vi "Apply Tombstone Target.vi"   [LabVIEW 2018, in "Toolkit.lvlib" / "Tests.lvlib"]
uses:
  Tests.lvlib
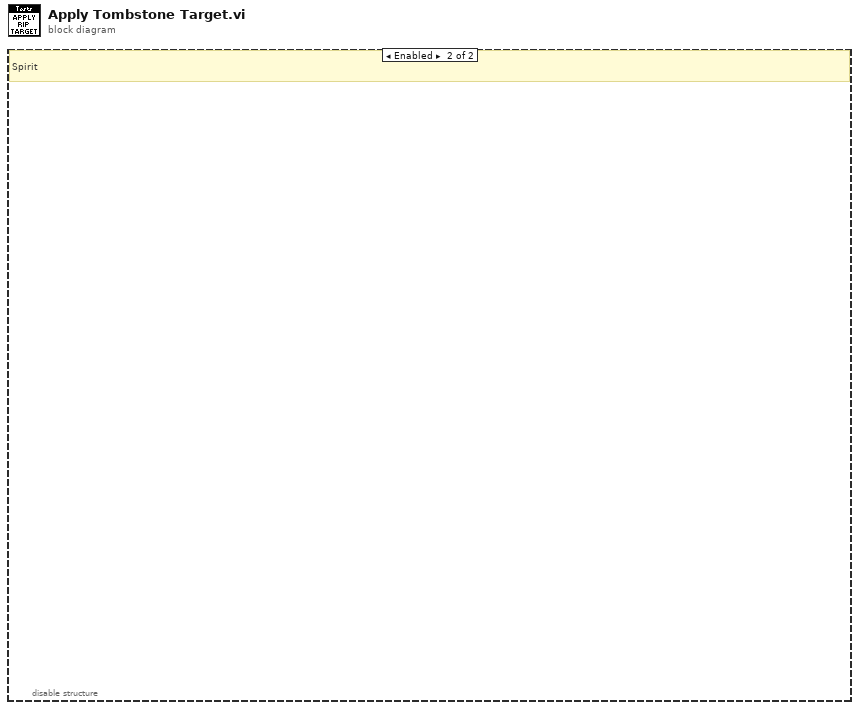
[diagram p0: block diagram]
diagram:
  n1 = disable-structure shown="Enabled" {
    frame Disabled {
      # "Corpse"
    }
    frame Enabled {
      # "Spirit"
    }
  }
